vi "package.vi"() -> ()   [LabVIEW 2024]
uses:
  Program Files (x86)/National Instruments/LabVIEW 2020/vi.lib/Maxon/emuCommands.lvlibp/schemas/SoftwareVersion.ctl
  Program Files (x86)/National Instruments/LabVIEW 2020/vi.lib/Maxon/emuCommunication.lvlibp/emuCommunication/emuCommunication.lvclass
  C:/Program Files (x86)/National Instruments/LabVIEW 2020/vi.lib/Maxon/emuInterfaces.lvlibp/iEmuCommunication/iEmuCommunication.lvclass
  Program Files (x86)/National Instruments/LabVIEW 2020/vi.lib/Maxon/emuCommands.lvlibp/cmdFactory/cmdFactory.lvclass
  Program Files (x86)/National Instruments/LabVIEW 2020/vi.lib/Maxon/emuInterfaces.lvlibp/iEmuCommand/iEmuCommand.lvclass
  Program Files (x86)/National Instruments/LabVIEW 2020/vi.lib/Maxon/emuCommands.lvlibp/commands/Misc/System/SoftwareVersion/Misc_System_SoftwareVersion.lvclass
  Program Files (x86)/National Instruments/LabVIEW 2020/vi.lib/Maxon/emuCommands.lvlibp
panel:
  out "ResponseData":T1
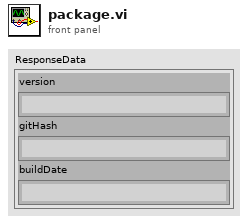
[diagram p1: front panel]
types:
  T1 = typedef "emuCommands.lvlibp/SoftwareVersion.ctl" = cluster{"version":string, "gitHash":string, "buildDate":string}
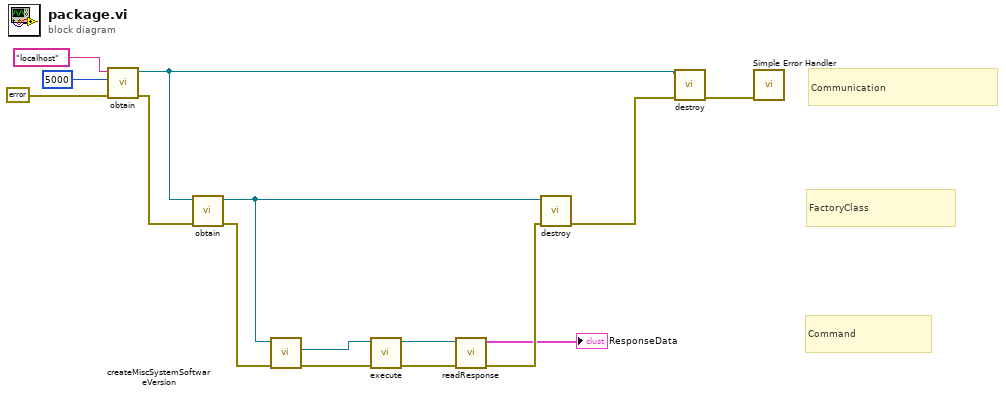
[diagram p0: block diagram]
diagram:
  # "Command"
  # "FactoryClass"
  # "Communication"
  n1 = call "obtain.vi"("error in (no error)"=errorcluster {"status"=FALSE, "code"=0, "source"=""}, "port"=5000, "address"="localhost") -> ("error out"=w8:errorcluster, "emuCommunication out"=w6:refnum<class "emuCommunication.lvclass">)  [unwired: 7 in]
  n2 = call "obtain.vi"("error in (no error)"=w8, "iEmuCommunication"=w6) -> ("error out"=w9:errorcluster, "emuCommandFactory out"=w10:refnum<class "cmdFactory.lvclass">)  [unwired: 8 in]
  n3 = call-dynamic "createMiscSystemSoftwareVersion.vi"("error in (no error)"=w9, "emuCommandFactory in"=w10) -> ("error out"=w14:errorcluster, "Misc_System_SoftwareVersion out"=w15:refnum<class "iEmuCommand.lvclass">)  [unwired: 8 in]
  n4 = call-dynamic "execute.vi"("error in (no error)"=w14, "iEmuCommand in"=w15) -> ("error out"=w13:errorcluster, "iEmuCommand out"=w12:refnum<class "iEmuCommand.lvclass">)  [unwired: 8 in]
  n5 = call "readResponse.vi"("error in (no error)"=w13, "Misc_System_SoftwareVersion in"=w12) -> ("error out"=w11:errorcluster, "ResponseData"=→"ResponseData":T1)  [unwired: 8 in]
  n6 = call "destroy.vi"("error in (no error)"=w11, "emuCommandFactory in"=w10) -> ("error out"=w7:errorcluster)  [unwired: 9 in]
  n7 = call-dynamic "destroy.vi"("error in (no error)"=w7, "emuCommunication in"=w6) -> ("error out"=w1:errorcluster)  [unwired: 9 in]
  n8 = call <vilib>:"Simple Error Handler.vi"("error in (no error)"=w1) -> ()  [unwired: 4 in, 5 out]
